vi "Write Device ID Type.vi"(8 "error in":errorcluster, 10 "device ID type":T1=1 items=["None"=0, "Basic Stream"=1, "Regular Stream"=2, "Extended Stream"=3, "Basic Stream/Individual"=129, "Regular Stream/Individual"=130, "Extended Stream/Individual"=131], 11 "device data model in":refnum<class "Device Data Model.lvclass">) -> (0 "error out":errorcluster, 3 "device data model out":refnum<class "Device Data Model.lvclass">)   [LabVIEW 2012, in "Device Data Model.lvclass"]
doc: "Writes the value of the device ID."
uses:
  Device Data Model.lvclass
  Device ID Type.ctl
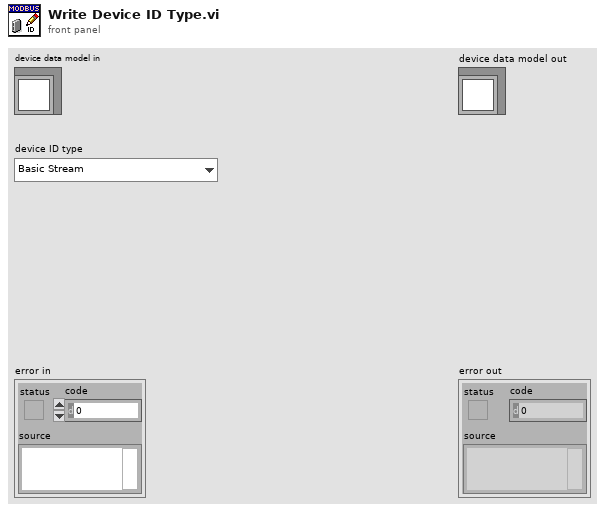
[diagram p1: front panel]
types:
  T1 = typedef "Device Data Model.lvclass/Device ID Type.ctl" = u8
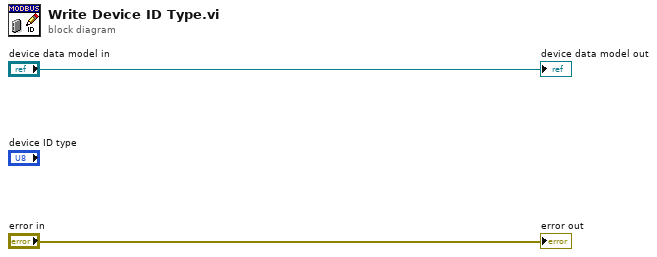
[diagram p0: block diagram]
diagram:
  "error out" <- "error in"
  "device data model out" <- "device data model in"
